vi "Broadcast Message.vi"(7 "Module Pattern (support *)":string, 8 "Error in":errorcluster caption="Error in (no error)", 10 "Argument(\"\")":string, 11 "Message":string) -> (0 "Error out":errorcluster)   [LabVIEW 2017, in "_csmlite.lvlib"]
uses:
  _csmlite.lvlib
  _action.ctl
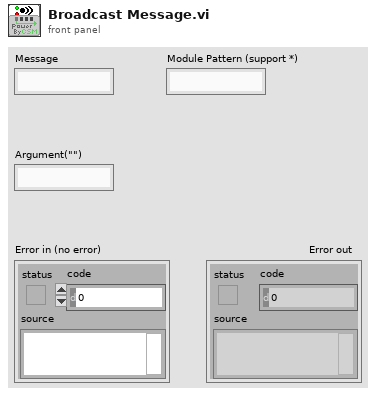
[diagram p1: front panel]
types:
  T1 = typedef "_csmlite.lvlib/_action.ctl" = enum16{"Obtain", "Destroy", "Broadcast", "Post", "List"}
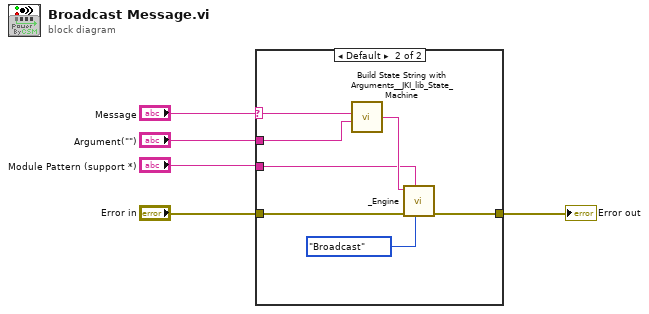
[diagram p0: block diagram]
diagram:
  n1 = case shown="Default" "Message" {
    selector: "Message" -> [_ w9]
    tunnel: "Error in" -> [w6 w12]
    tunnel: [w6 w11] -> w4
    tunnel: "Argument(\"\")" -> [_ w8]
    tunnel: "Module Pattern (support *)" -> [_ w7]
    frame "" {
    }
    frame Default {
      n2 = call <vilib>:"Build State String with Arguments__JKI_lib_State_Machine.vi"("Arguments (\"\")"=w8, "State"=w9) -> ("State with Arguments"=w10:string)  [unwired: 4 in]
      n3 = call "_Engine.vi"("Enum"=_action."Broadcast", "Module Name"=w7, "Error in"=w12, "Message"=w10) -> ("Error out"=w11:errorcluster)  [unwired: 5 in, 2 out]
    }
  }
  "Error out" <- w4
